vi "Get_FrameRate.vi"(8 "error in (no error)":errorcluster, 11 "Avantes in":refnum<class "Avantes.lvclass">) -> (0 "error out":errorcluster, 2 "Frame Rate":dbl[unit], 3 "Avantes out":refnum<class "Avantes.lvclass">)   [LabVIEW 2020, in "Avantes.lvclass"]
uses:
  <instrlib>/Classes/CCD/Avantes/Avantes.lvclass
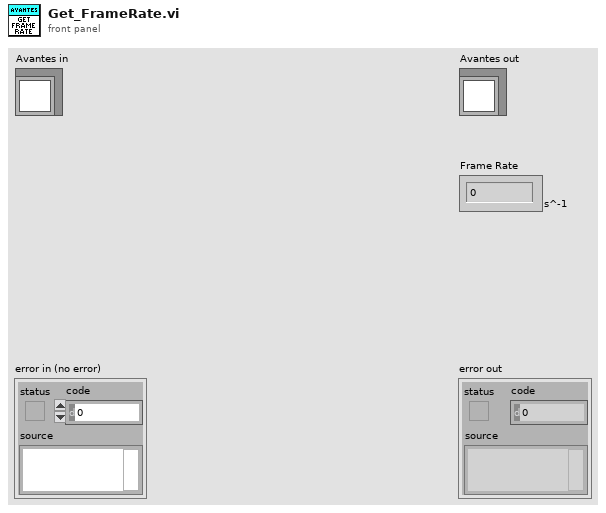
[diagram p1: front panel]
types:
  T1 = typedef "clusterdef.ctl" = cluster{"Len":u16, "ConfigVersion":u16, "UserFriendlyId":u8[], "DetectorType":cluster{"SensorType":u8, "NrPixels":u16, "Fit":sgl[], "NLEnable":u8, "NLCorrect":dbl[], "LowNLCounts":dbl, "HighNLCounts":dbl, "Gain":sgl[], "Reserved":sgl, "Offset":sgl[], "Extern Offset":sgl, "DefectivePixels":u16[]}, "IrradianceType":cluster{"SpectrumCalibrationType":cluster{"SmoothingType":cluster{"m_SmoothPix":u16, "SmoothModel":u8}, "CalInttime":sgl, "CalibConvers":sgl[]}, "CalibrationType":u8, "FiberDiameter":i32}, "SpectrumCalibrationType":cluster{"SmoothingType":cluster{"m_SmoothPix":u16, "SmoothModel":u8}, "CalInttime":sgl, "CalibConvers":sgl[]}, "SpectrumCorrectionType":sgl[], "StandAloneType":cluster{"StandAloneType":u8, "MeasConfigType":cluster{"StartPixel":u16, "StopPixel":u16, "IntegrationTime":sgl, "IntegrationDelay":u32, "NrAverages":u32, "DarkCorrectionType":cluster{"Enable CorDynDark":u8, "ForgetPercentage":u8}, "SmoothingType":cluster{"SmoothPix":u16, "SmoothModel":u8}, "SatDetection":u8, "TriggerType":cluster{"Trigger Mode":u8, "Trigger Source":u8, "Trigger SourceType":u8}, "ControlSettingsType":cluster{"StrobeControl":u16, "LaserDelay":u32, "LaserWidth":u32, "LaserWaveLength":sgl, "StoreToRam":u16}}, "Nmsr":i16}, "DynamicStorageType":cluster{"Nmsr":i32, "Reserved":u8[]}, "TempSensorType":sgl[], "TecControlType":cluster{"Enable":u8, "Setpoint":sgl, "Fit[NR_DAC_POL_COEF]":sgl[]}, "ProcessControlType":cluster{"AnalogLow":sgl[], "AnalogHigh":sgl[], "DigitalLow":sgl[], "DigitalHigh":sgl[]}, "EthernetSettingsType":cluster{"IpAddr":u32, "NetMask":u32, "Gateway":u32, "DhcpEnabled":u8, "TcpPort":u16, "LinkStatus":u8}, "Reserved":u8[], "OemData":u8[]}
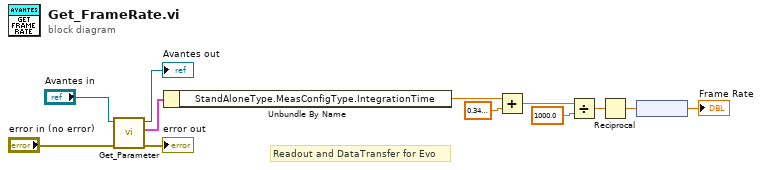
[diagram p0: block diagram]
diagram:
  # "Readout and DataTransfer for Evo"
  n1 = call-dynamic "Get_Parameter.vi"("error in (no error)"="error in (no error)", "Avantes in"="Avantes in") -> ("error out"=→"error out":errorcluster, "DeviceConfig"=w8:T1, "Avantes out"=→"Avantes out":refnum<class "Avantes.lvclass">)  [unwired: 7 in]
  n2 = Unbundle By Name(w8) -> ("StandAloneType.MeasConfigType.IntegrationTime"=w7:sgl)
  n3 = Add(x=w7, y=sgl 0.35) -> (x+y=w5:sgl)
  n4 = Divide(x=w5, y=sgl 1000.0) -> (x/y=w3:sgl)
  n5 = Reciprocal(x=w3) -> (1/x=w2:sgl)
  n6 = node(w2) -> (→"Frame Rate":sgl[unit])
